vi "SenalAnchoBanda.vi"(2 "Puntos a generar-chirp":i32=100, 3 "Rango Frec para chrip":cluster{"start freq":dbl, "end freq":dbl}={"start freq"=0.5, "end freq"=2.0} {"end freq" format="%0.2f"; "start freq" format="%0.2f"}, 4 "Tm":dbl=0.02, 5 "Zona muerta":dbl=0.2, 6 "amplitude":dbl=0.1 format="%0.2f", 7 "Señal a generar":enum16{"Chirp", "Archivo"}(ring)=enum."Archivo") -> (0 "offset":dbl, 1 "Señal":dbl[](array[numeric]))   [LabVIEW 2013]
uses:
  <vilib>/measure/maspectr.llb/FFT Spectrum (Mag-Phase) for 1 Chan.vi
  <vilib>/Analysis/NI_AALBase.lvlib
  <vilib>/measure/NI_MAPro.lvlib
panel:
  in  "file path (dialog if empty) 2":path=path "C:/tiempo.txt"
  out "array":dbl[][](array[numeric]) format="%#_9g"
  in  "file path (dialog if empty)":path=path "C:/Amplitud.txt"
  out "Tiempo de ejecución chrp":dbl
  out "spectrum units table":string[][](table)=[["FFT", "N * V", "N/2 * Vpk"], ["Power Spectrum", "V^2", "1/2 * Vrms^2"], ["Auto Power Spectrum", "V^2", "Vrms^2"], ["Amplitude and Phase Spectrum", "V", "Vrms"], ["FFT Power Spectrum", "V^2", "Vrms^2"], ["FFT Power Spectral Density", "V^2/Hz", "Vrms^2/Hz"], ["FFT Spectrum (Mag-Phase)", "V", "Vrms"], ["FFT Spectrum (Real-Imag)", "V", "Vrms"]]
  out "max index(es)":i32
  out "Max freq":dbl
  out "max frec value":dbl
  out "FFT":waveform(dbl)(graph)
  out "df":dbl
  out "f0":dbl
  out "Señal":waveform(dbl)(graph)
  out "Clck Rate":dbl
  # "Chirp"
  # "df (Hz) = Fs/N"
  # "Vrms=Vpico*0,707"
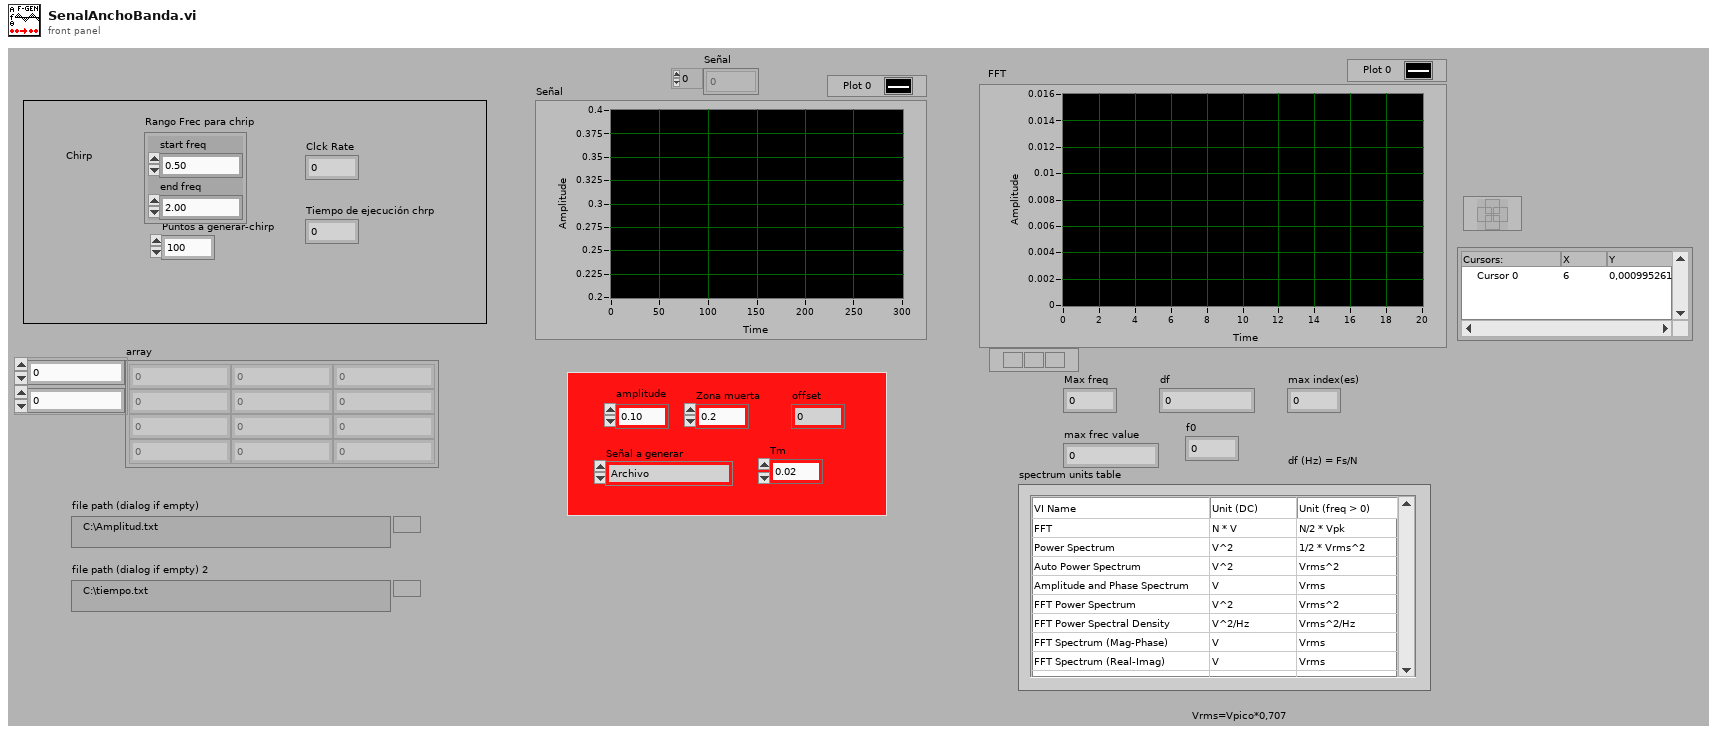
[diagram p1: front panel]
types:
  T1 = enum16{"None ", "Hanning", "Hamming", "Blackman-Harris", "Exact Blackman", "Blackman", "Flat Top", "4 Term B-Harris ", "7 Term B-Harris", "Low Sidelobe"}
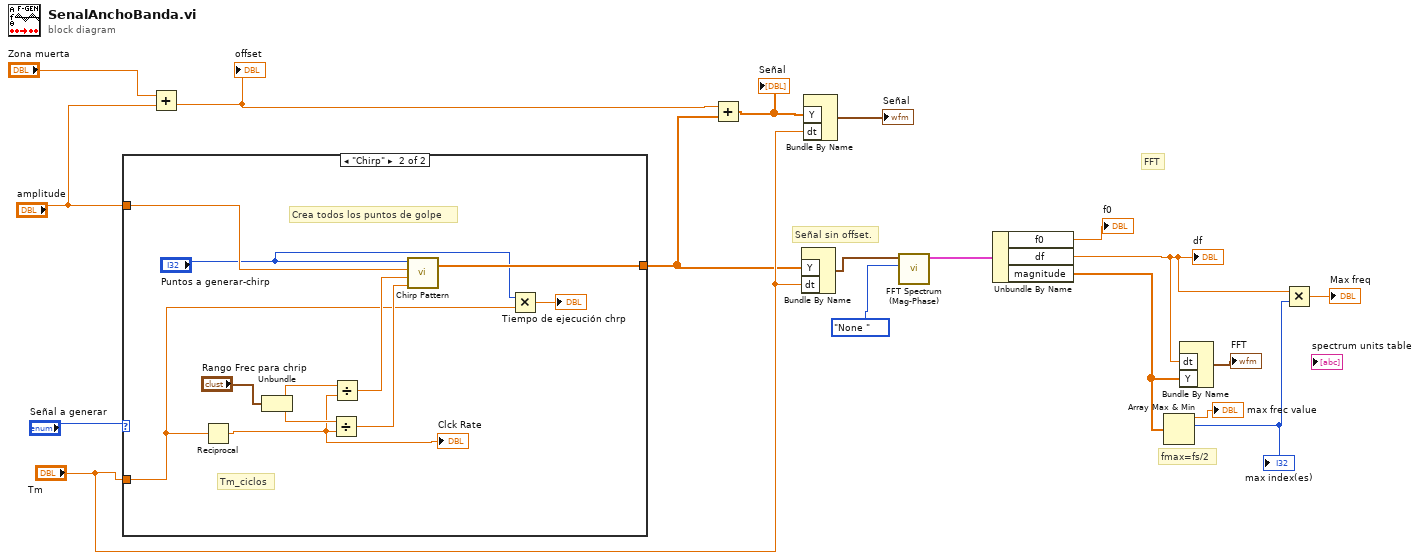
[diagram p0: block diagram]
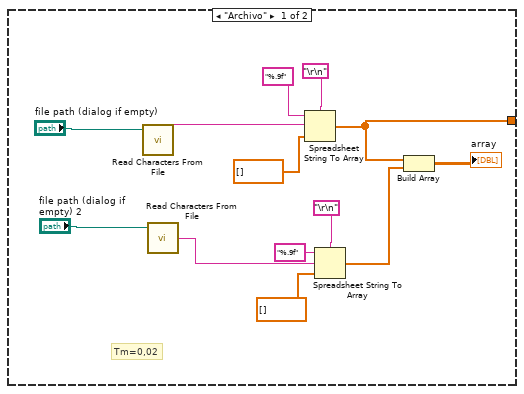
[diagram p2: hidden frame]
diagram:
  # "FFT"
  # "Señal sin offset."
  # "fmax=fs/2"
  n1 = case shown="\"Chirp\"" "Señal a generar" {
    tunnel: "amplitude" -> [_ w42]
    tunnel: [w19 w41] -> w4
    tunnel: "Tm" -> [_ w33]
    frame "Archivo" {
      # "Tm=0,02"
      n2 = call <vilib>:"Read Characters From File.vi"("file path (dialog if empty)"="file path (dialog if empty)") -> ("character string"=w28:string)  [unwired: 5 in, 3 out]
      n3 = call <vilib>:"Read Characters From File.vi"("file path (dialog if empty)"="file path (dialog if empty) 2") -> ("character string"=w24:string)  [unwired: 5 in, 3 out]
      n4 = Spreadsheet String To Array(delimiter (Tab)="\r\n", format string="%.9f", spreadsheet string=w28, array type (2D Dbl)=dbl[] []) -> (array=w19:dbl[])
      n5 = Spreadsheet String To Array(delimiter (Tab)="\r\n", format string="%.9f", spreadsheet string=w24, array type (2D Dbl)=dbl[] []) -> (array=w23:dbl[])
      n6 = Build Array(w19, w23) -> (→"array":dbl[][])
    }
    frame "Chirp" {
      # "Tm_ciclos"
      # "Crea todos los puntos de golpe"
      n7 = Reciprocal(x=w33) -> (1/x=w35:dbl)
      "Clck Rate" <- w35
      n8 = Unbundle("Rango Frec para chrip") -> ("start freq"=w39:dbl, "end freq"=w40:dbl)
      n9 = Divide(x=w40, y=w35) -> (x/y=w36:dbl)
      n10 = Divide(x=w39, y=w35) -> (x/y=w37:dbl)
      n11 = call <vilib>:"Chirp Pattern.vi"("f2"=w36, "f1"=w37, "amplitude"=w42, "samples"="Puntos a generar-chirp") -> ("Chirp Pattern"=w41:dbl[])  [unwired: 1 out]
      n12 = Multiply(x="Puntos a generar-chirp", y=w33) -> (x*y=→"Tiempo de ejecución chrp":dbl)
    }
  }
  n13 = Add(x="Zona muerta", y="amplitude") -> (x+y=w8:dbl)
  "offset" <- w8
  n14 = Add(x=w8, y=w4) -> (x+y=w5:dbl[])
  "Señal" <- w5
  n15 = Bundle By Name("Y"=w4, "dt"="Tm") -> (w6:waveform(dbl))  [unwired: 1 in]
  n16 = Bundle By Name("Y"=w5, "dt"="Tm") -> (→"Señal":waveform(dbl))  [unwired: 1 in]
  n17 = call-poly <vilib>:"FFT Spectrum (Mag-Phase).vi"("window"=T1."None ", "time signal"=w6) -> ("magnitude"=w16:cluster{"f0":dbl, "df":dbl, "magnitude":dbl[]})  [unwired: 5 in, 4 out]
  n18 = Unbundle By Name(w16) -> ("f0"=→"f0":dbl, "df"=w2:dbl, "magnitude"=w1:dbl[])
  "df" <- w2
  n19 = Array Max & Min(array=w1) -> (max value=→"max frec value":dbl, max index (indices)=w12:i32)  [unwired: 2 out]
  "max index(es)" <- w12
  n20 = Bundle By Name("dt"=w2, "Y"=w1) -> (→"FFT":waveform(dbl))  [unwired: 1 in]
  n21 = Multiply(x=w2, y=w12) -> (x*y=→"Max freq":dbl)
